vi "Write UserDefined State.vi"(8 "error in (no error)":errorcluster, 10 "state":refnum<class "state.lvclass">, 11 "user-defined-state in":refnum<class "user-defined-state.lvclass">) -> (0 "error out":errorcluster, 3 "user-defined-state out":refnum<class "user-defined-state.lvclass">)   [LabVIEW 2020, in "eos.lvlib" / "user-defined-state.lvclass"]
uses:
  user-defined-state.lvclass
  interfaces/state/state.lvclass
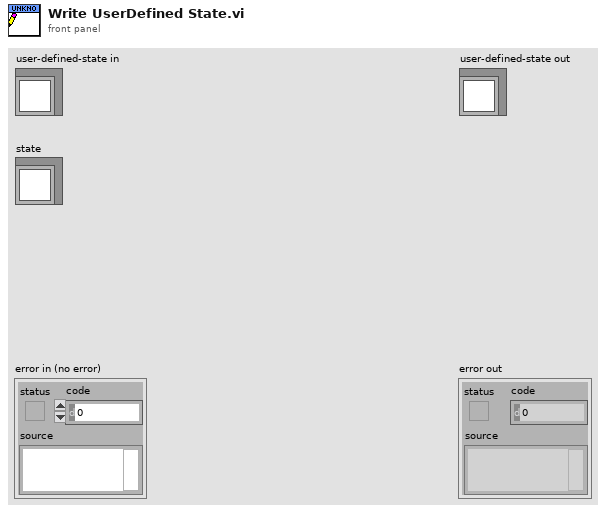
[diagram p1: front panel]
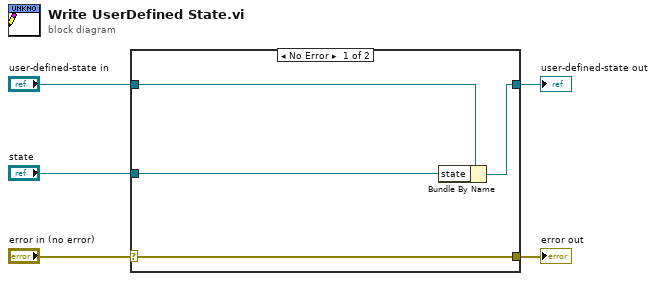
[diagram p0: block diagram]
diagram:
  n1 = case shown="No Error" "error in (no error)" {
    selector: "error in (no error)" -> [w9 w10]
    tunnel: [w9 w10] -> w4
    tunnel: [w7 w11] -> w2
    tunnel: "user-defined-state in" -> [w8 w11]
    tunnel: "state" -> [w6 _]
    frame No Error {
      n2 = Bundle By Name(cluster=w8, "state"=w6) -> (w7:refnum<class "user-defined-state.lvclass">)
    }
    frame Error {
    }
  }
  "error out" <- w4
  "user-defined-state out" <- w2
